vi "String Constant - Inside Nested Case Structure.vi"() -> ()   [LabVIEW 2020]
panel:
  in  "OK":bool
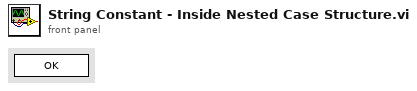
[diagram p1: front panel]
types:
  T1 = enum32{"Invalid", "Standard", "Closed", "Hidden", "Minimized", "Maximized"}
  T2 = enum32{"invalid app kind", "Development System", "Run Time System", "Student Edition", "Embedded LabVIEW", "Evaluation", "Custom"}
  T3 = cluster{"Core":cluster{"Current VI Reference":refnum<vi>, "Close Panel on Exit?":bool}, "Your Boolean data":bool}
  T4 = cluster{"Current VI Reference":refnum<vi>, "Close Panel on Exit?":bool}
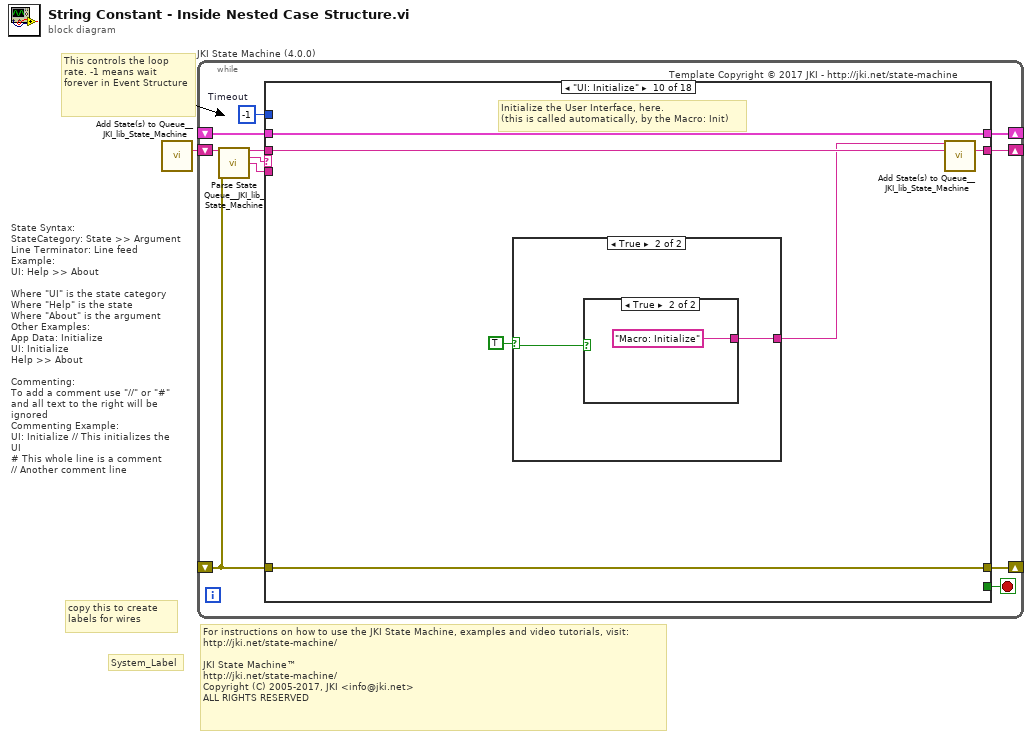
[diagram p0: block diagram]
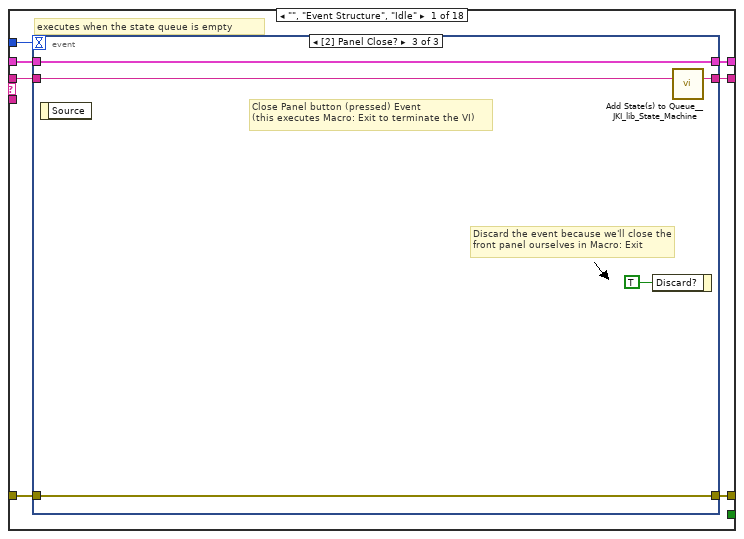
[diagram p2: hidden frame]
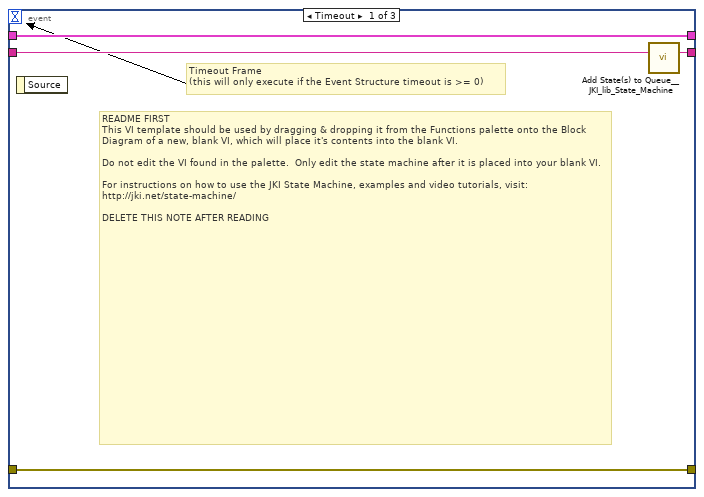
[diagram p3: hidden frame]
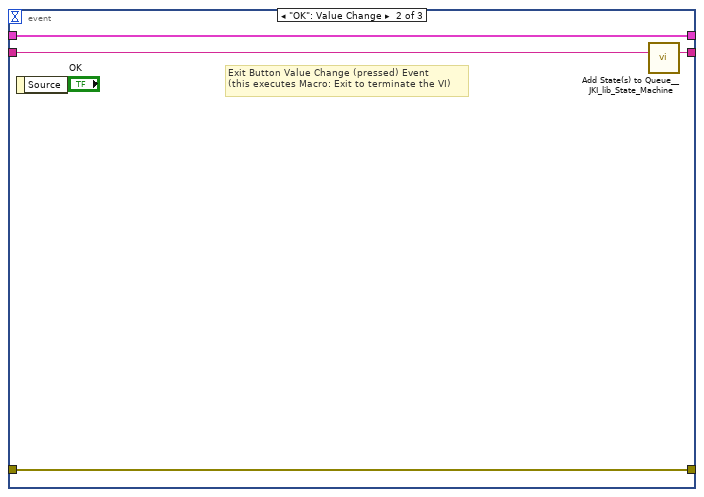
[diagram p4: hidden frame]
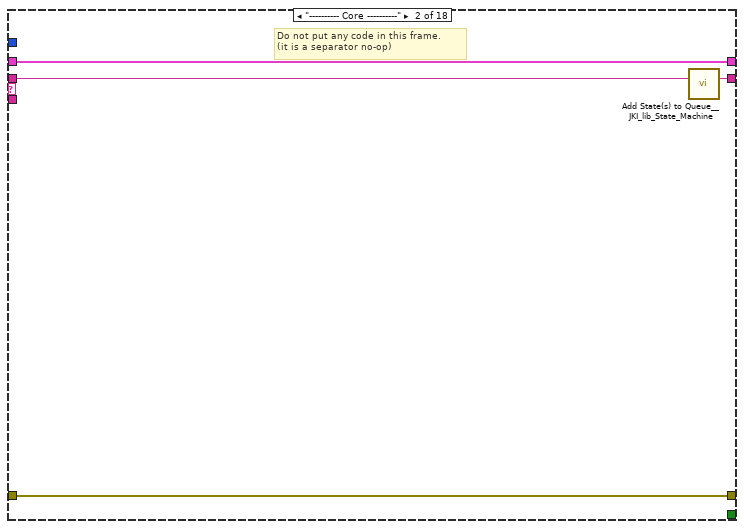
[diagram p5: hidden frame]
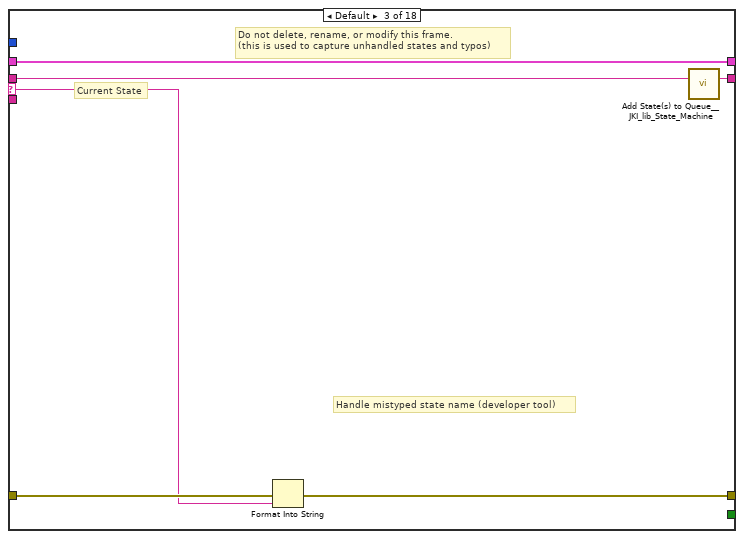
[diagram p6: hidden frame]
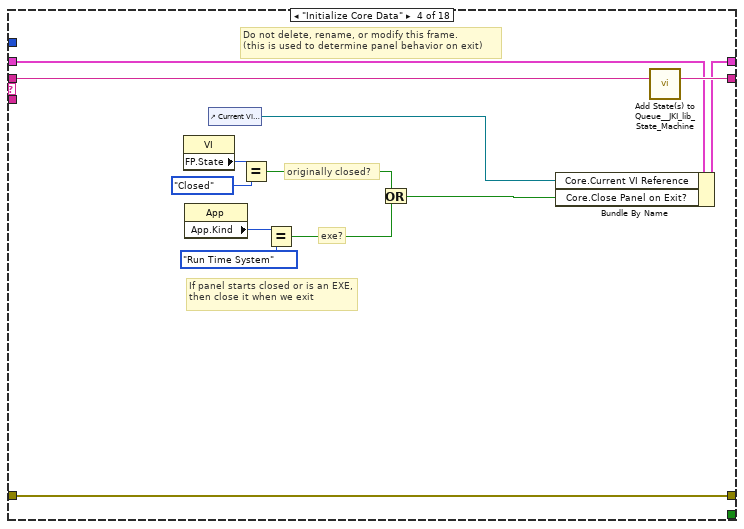
[diagram p7: hidden frame]
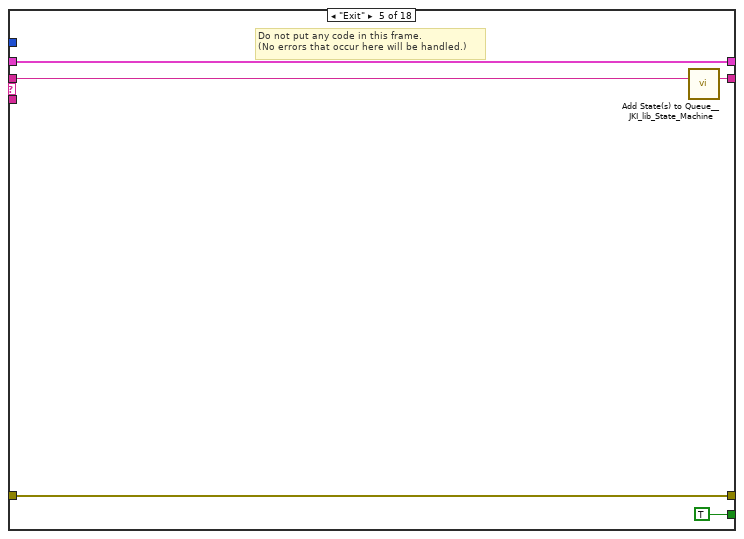
[diagram p8: hidden frame]
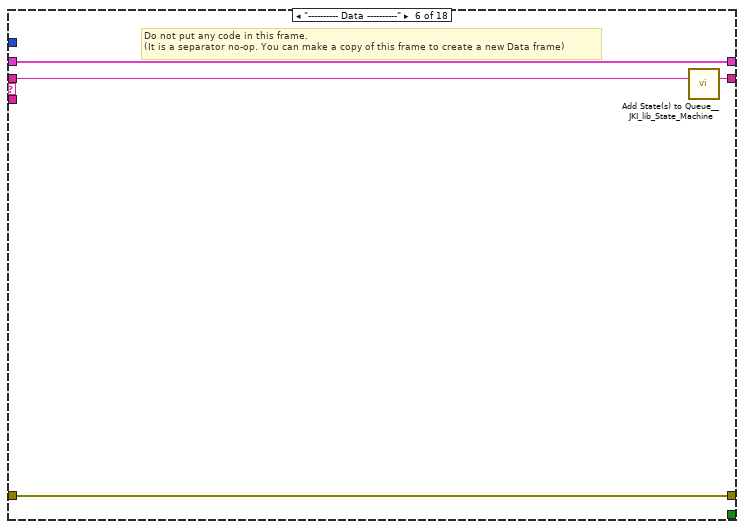
[diagram p9: hidden frame]
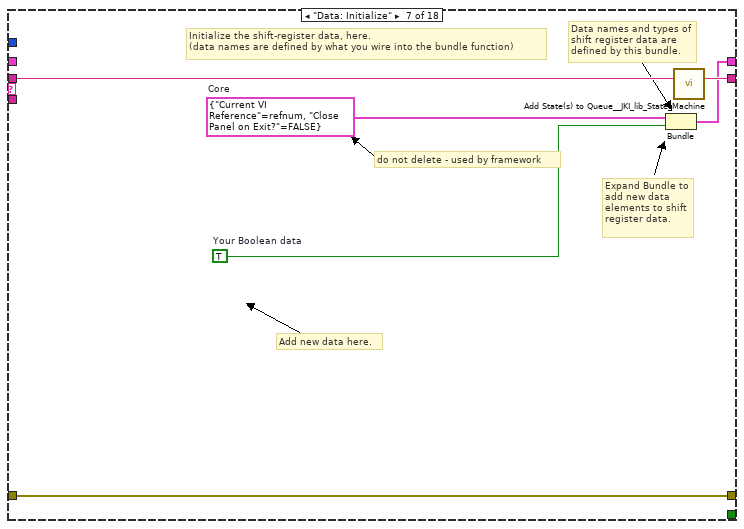
[diagram p10: hidden frame]
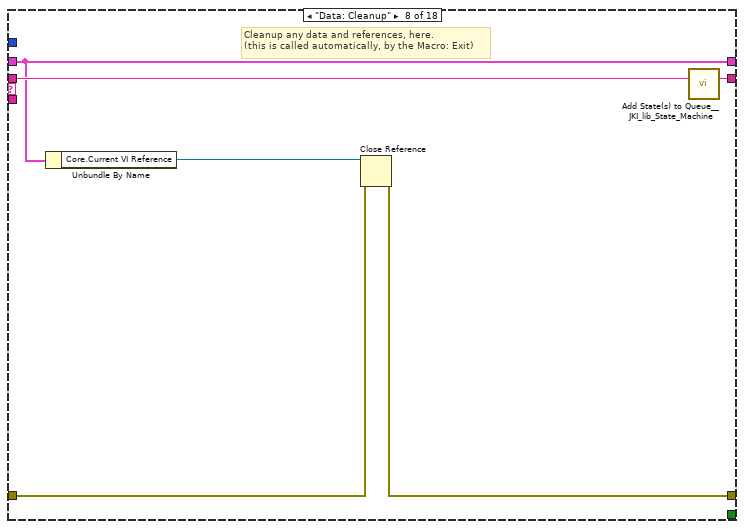
[diagram p11: hidden frame]
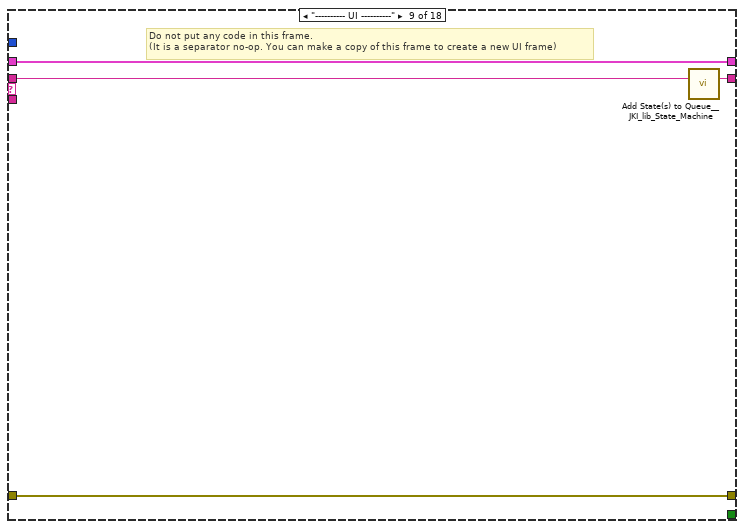
[diagram p12: hidden frame]
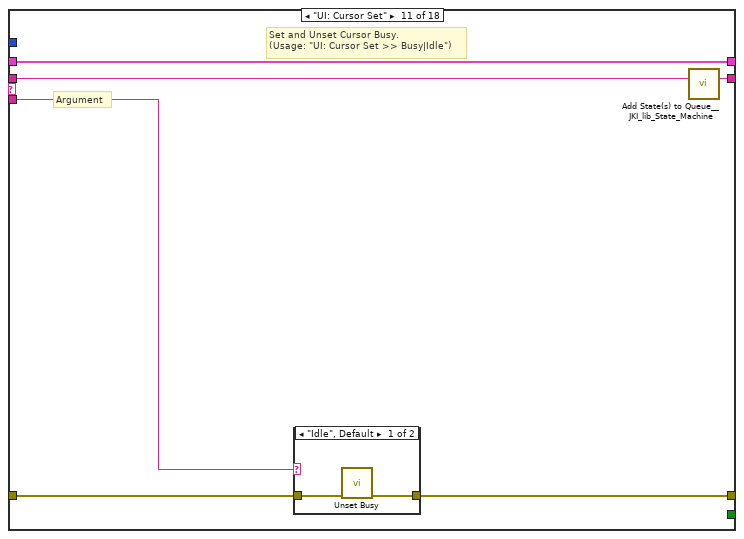
[diagram p15: hidden frame]
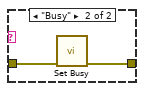
[diagram p16: hidden frame]
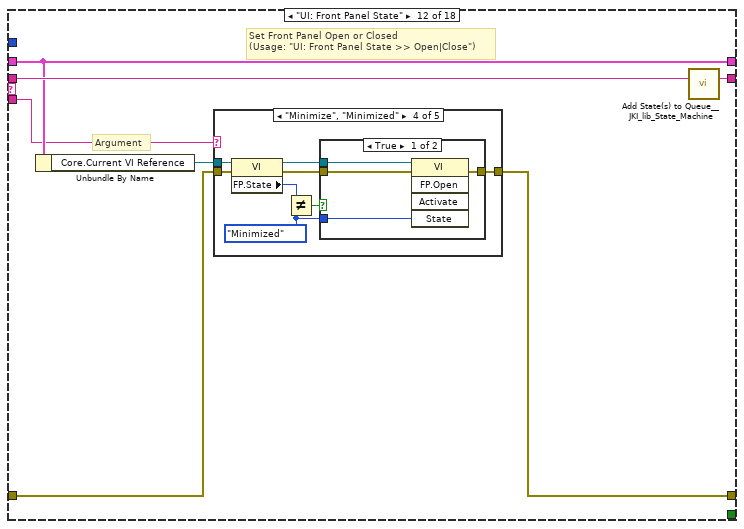
[diagram p17: hidden frame]
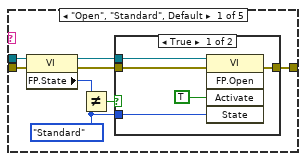
[diagram p18: hidden frame]
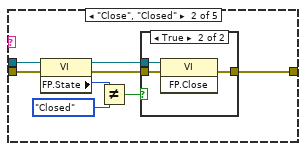
[diagram p20: hidden frame]
diagram:
  # "For instructions on how to use the JKI State Machine, examples and video tutorials, visit:\nhttp://jki.net/state-machine/\n\nJKI State Machine™\nhttp://jki.net/state-machine/\nCopyright (C) 2005-2017, JKI <info@jki.net>\nALL RIGHTS RESERVED"
  # "State Syntax:\nStateCategory: State >> Argument\nLine Terminator: Line feed\nExample:\nUI: Help >> About\n\nWhere \"UI\" is the state category\nWhere \"Help\" is the state\nWhere \"About\" is the argument\nOther Examples:\nApp Data: Initialize\nUI: Initialize\nHelp >> About\n\nCommenting:\nTo add a comment use \"//\" or \"#\" and all text to the right will be ignored\nCommenting Example:\nUI: Initialize // This initializes the UI\n# This whole line is a comment\n// Another comment line"
  # "copy this to create labels for wires"
  # "This controls the loop rate. -1 means wait forever in Event Structure"
  # "System_Label"
  n1 = call <vilib>:"Add State(s) to Queue__JKI_lib_State_Machine.vi"() -> ("States Out"=w1:string)  [unwired: 15 in]
  n2 = while "JKI State Machine (4.0.0)" {
    shift-right: [w5] -> _
    shift-left: _ -> [w4]
    shift-right: [w8] -> _
    shift-left: _ -> [w2]
    shift-right: [w7] -> _
    shift-left: w1 -> [w9]
    stop <- w6 stop-if-true
    w3 = -1  # Timeout
    # "Template Copyright © 2017 JKI - http://jki.net/state-machine"
    n3 = call <vilib>:"Parse State Queue__JKI_lib_State_Machine.vi"("State Queue"=w9, "Error In (no error)"=w2) -> ("Remaining States"=w11:string, "Current State"=w12:string, "Arguments"=w10:string)  [unwired: 11 in]
    n4 = case shown="\"UI: Initialize\"" w12 {
      selector: w12 -> [_ _ w37 _ _ _ _ _ _ _ _ _ _ _ _ _ _ _]
      tunnel: w11 -> [w19 w36 w40 w55 w60 w64 w70 w76 w80 w86 w95 w106 w175 w179 w183 w187 w191 w195]
      tunnel: w10 -> [_ _ _ _ _ _ _ _ _ _ w90 w100 _ _ _ _ _ _]
      tunnel: w4 -> [w17 w33 w38 w48 w58 w61 _ w71 w77 w84 w93 w102 w172 w176 w180 w184 w188 w192]
      tunnel: [w16 w34 w42 w52 w57 w62 w67 w72 w78 w83 w91 w103 w173 w177 w181 w185 w189 w193] -> w8
      tunnel: w2 -> [w15 w34 w41 w52 w57 w62 w67 w73 w78 w83 w92 w104 w173 w177 w181 w185 w189 w193]
      tunnel: [w18 w35 w39 w54 w59 w63 w69 w75 w79 w85 w94 w105 w174 w178 w182 w186 w190 w194] -> w7
      tunnel: [_ _ _ _ TRUE _ _ _ _ _ _ _ _ _ _ _ _ _] -> w6
      tunnel: [w14 w33 w38 w53 w58 w61 w68 w71 w77 w84 w93 w102 w172 w176 w180 w184 w188 w192] -> w5
      tunnel: w3 -> [w13 _ _ _ _ _ _ _ _ _ _ _ _ _ _ _ _ _]
      frame "", "Event Structure", "Idle" {
        # "executes when the state queue is empty"
        n5 = event shown="[2] Panel Close?" {
          selector: _ -> [_ _ _]
          dyn-events: _ -> [_ _ _]
          timeout: w13 -> [_ _ _]
          tunnel: w19 -> [w23 w27 w32]
          tunnel: [w22 w26 w31] -> w18
          tunnel: w17 -> [w20 w24 w29]
          tunnel: [w21 w25 w30] -> w16
          tunnel: w15 -> [w21 w25 w30]
          tunnel: [w20 w24 w29] -> w14
          event Timeout {
            # "README FIRST\nThis VI template should be used by dragging & dropping it from the Functions palette onto the Block Diagram of a new, blank VI, which will place it's contents into the blank VI.\n\nDo not edit the VI found in the palette.  Only edit the state machine after it is placed into your blank VI.\n\nFor instructions on how to use the JKI State Machine, examples and video tutorials, visit:\nhttp://jki.net/state-machine/\n\nDELETE THIS NOTE AFTER READING"
            # "Timeout Frame\n(this will only execute if the Event Structure timeout is >= 0)"
            n6 = event-data() -> ()  [unwired: 1 in, 1 out]
            n7 = call <vilib>:"Add State(s) to Queue__JKI_lib_State_Machine.vi"("State(s) in (\"\")"=w23) -> ("States Out"=w22:string)  [unwired: 14 in]
          }
          event "OK": Value Change {
            # "Exit Button Value Change (pressed) Event\n(this executes Macro: Exit to terminate the VI)"
            n8 = event-data() -> ()  [unwired: 1 in, 1 out]
            n9 = call <vilib>:"Add State(s) to Queue__JKI_lib_State_Machine.vi"("State(s) in (\"\")"=w27) -> ("States Out"=w26:string)  [unwired: 14 in]
          }
          event Panel Close? {
            # "Discard the event because we'll close the front panel ourselves in Macro: Exit"
            # "Close Panel button (pressed) Event\n(this executes Macro: Exit to terminate the VI)"
            n10 = event-data() -> ()  [unwired: 1 in, 1 out]
            n11 = event-data("Discard?"=TRUE) -> ()  [unwired: 1 in, 1 out]
            n12 = call <vilib>:"Add State(s) to Queue__JKI_lib_State_Machine.vi"("State(s) in (\"\")"=w32) -> ("States Out"=w31:string)  [unwired: 14 in]
          }
        }
      }
      frame "---------- Core ----------" {
        # "Do not put any code in this frame.\n(it is a separator no-op)"
        n13 = call <vilib>:"Add State(s) to Queue__JKI_lib_State_Machine.vi"("State(s) in (\"\")"=w36) -> ("States Out"=w35:string)  [unwired: 14 in]
      }
      frame Default {
        # "Current State"
        # "Do not delete, rename, or modify this frame.\n(this is used to capture unhandled states and typos)"
        # "Handle mistyped state name (developer tool)"
        n14 = Format Into String(error in=w41, w37) -> (error out=w42:errorcluster)  [unwired: 2 in, 1 out]
        n15 = call <vilib>:"Add State(s) to Queue__JKI_lib_State_Machine.vi"("State(s) in (\"\")"=w40) -> ("States Out"=w39:string)  [unwired: 14 in]
      }
      frame "Initialize Core Data" {
        # "Do not delete, rename, or modify this frame.\n(this is used to determine panel behavior on exit)"
        # "originally closed?"
        # "exe?"
        # "If panel starts closed or is an EXE, then close it when we exit"
        n16 = property class="VI"() -> ("FP.State"=w45:T1)  [unwired: 2 in, 2 out]
        n17 = property class="App"() -> ("App.Kind"=w51:T2)  [unwired: 2 in, 2 out]
        n18 = control-ref of="Current VI Reference"() -> (w46:refnum<vi>)
        n19 = Equal?(x=w45, y=T1."Closed" ("Front Panel Window:State")) -> (x = y?=w43:bool)
        n20 = Equal?(x=w51, y=T2."Run Time System" ("Application:Kind")) -> (x = y?=w49:bool)
        n21 = Or(x=w43, y=w49) -> (x .or. y?=w47:bool)
        n22 = Bundle By Name(cluster=w48, "Core.Current VI Reference"=w46, "Core.Close Panel on Exit?"=w47) -> (w53:T3)
        n23 = call <vilib>:"Add State(s) to Queue__JKI_lib_State_Machine.vi"("State(s) in (\"\")"=w55) -> ("States Out"=w54:string)  [unwired: 14 in]
      }
      frame "Exit" {
        # "Do not put any code in this frame.\n(No errors that occur here will be handled.)"
        n24 = call <vilib>:"Add State(s) to Queue__JKI_lib_State_Machine.vi"("State(s) in (\"\")"=w60) -> ("States Out"=w59:string)  [unwired: 14 in]
      }
      frame "---------- Data ----------" {
        # "Do not put any code in this frame.\n(It is a separator no-op. You can make a copy of this frame to create a new Data frame)"
        n25 = call <vilib>:"Add State(s) to Queue__JKI_lib_State_Machine.vi"("State(s) in (\"\")"=w64) -> ("States Out"=w63:string)  [unwired: 14 in]
      }
      frame "Data: Initialize" {
        w65 = T4 {"Current VI Reference"=refnum, "Close Panel on Exit?"=FALSE}  # Core
        w66 = TRUE  # Your Boolean data
        # "do not delete - used by framework"
        # "Expand Bundle to add new data elements to shift register data."
        # "Add new data here."
        # "Data names and types of shift register data are defined by this bundle."
        # "Initialize the shift-register data, here.\n(data names are defined by what you wire into the bundle function)"
        n26 = Bundle("Core"=w65, "Your Boolean data"=w66) -> (w68:T3)  [unwired: 1 in]
        n27 = call <vilib>:"Add State(s) to Queue__JKI_lib_State_Machine.vi"("State(s) in (\"\")"=w70) -> ("States Out"=w69:string)  [unwired: 14 in]
      }
      frame "Data: Cleanup" {
        # "Cleanup any data and references, here.\n(this is called automatically, by the Macro: Exit)"
        n28 = Unbundle By Name(w71) -> ("Core.Current VI Reference"=w74:refnum<vi>)
        n29 = Close Reference(reference=w74, error in (no error)=w73) -> (error out=w72:errorcluster)
        n30 = call <vilib>:"Add State(s) to Queue__JKI_lib_State_Machine.vi"("State(s) in (\"\")"=w76) -> ("States Out"=w75:string)  [unwired: 14 in]
      }
      frame "---------- UI ----------" {
        # "Do not put any code in this frame.\n(It is a separator no-op. You can make a copy of this frame to create a new UI frame)"
        n31 = call <vilib>:"Add State(s) to Queue__JKI_lib_State_Machine.vi"("State(s) in (\"\")"=w80) -> ("States Out"=w79:string)  [unwired: 14 in]
      }
      frame "UI: Initialize" {
        # "Initialize the User Interface, here.\n(this is called automatically, by the Macro: Init)"
        n32 = case shown="True" TRUE {
          selector: TRUE -> [_ w87]
          tunnel: [_ w88] -> w82
          frame False {
          }
          frame True {
            n33 = case shown="True" w87 {
              tunnel: [_ "Macro: Initialize"] -> w88
              frame False {
              }
              frame True {
              }
            }
          }
        }
        n34 = call <vilib>:"Add State(s) to Queue__JKI_lib_State_Machine.vi"("State(s) in Front (\"\")"=w82, "State(s) in (\"\")"=w86) -> ("States Out"=w85:string)  [unwired: 13 in]
      }
      frame "UI: Cursor Set" {
        # "Argument"
        # "Set and Unset Cursor Busy.\n(Usage: \"UI: Cursor Set >> Busy|Idle\")"
        n35 = case shown="\"Idle\", Default" w90 {
          tunnel: w92 -> [w97 w99]
          tunnel: [w96 w98] -> w91
          frame "Idle", Default {
            n36 = call <vilib>:"Unset Busy.vi"("error in (no error)"=w97) -> ("error out"=w96:errorcluster)  [unwired: 10 in]
          }
          frame "Busy" {
            n37 = call <vilib>:"Set Busy.vi"("error in (no error)"=w99) -> ("error out"=w98:errorcluster)  [unwired: 9 in, 1 out]
          }
        }
        n38 = call <vilib>:"Add State(s) to Queue__JKI_lib_State_Machine.vi"("State(s) in (\"\")"=w95) -> ("States Out"=w94:string)  [unwired: 14 in]
      }
      frame "UI: Front Panel State" {
        # "Argument"
        # "Set Front Panel Open or Closed\n(Usage: \"UI: Front Panel State >> Open|Close\")"
        n39 = Unbundle By Name(w102) -> ("Core.Current VI Reference"=w101:refnum<vi>)
        n40 = case shown="\"Minimize\", \"Minimized\"" w100 {
          tunnel: w104 -> [w112 w127 w138 w151 w164]
          tunnel: [w114 w128 w140 w153 w166] -> w103
          tunnel: w101 -> [w113 w125 w139 w152 w165]
          frame "Open", "Standard", Default {
            w107 = T1."Standard" ("State")
            n41 = property class="VI"(reference=w113, error in=w112) -> (reference out=w110:refnum<vi>, error out=w111:errorcluster, "FP.State"=w109:T1)
            n42 = Not Equal?(x=w109, y=w107) -> (x != y?=w108:bool)
            n43 = case shown="True" w108 {
              tunnel: [w118 w120] -> w114
              tunnel: w111 -> [w117 w120]
              tunnel: w110 -> [w116 _]
              tunnel: w107 -> [w115 _]
              frame True {
                n44 = invoke class="VI" method="FP.Open"(reference=w116, error in=w117, "Activate"=TRUE, "State"=w115) -> (error out=w118:errorcluster)  [unwired: 1 in, 4 out]
              }
              frame False {
              }
            }
          }
          frame "Close", "Closed" {
            n45 = property class="VI"(reference=w125, error in=w127) -> (reference out=w124:refnum<vi>, error out=w126:errorcluster, "FP.State"=w122:T1)
            n46 = Not Equal?(x=w122, y=T1."Closed" ("Front Panel Window:State")) -> (x != y?=w121:bool)
            n47 = case shown="True" w121 {
              tunnel: [w129 w132] -> w128
              tunnel: w126 -> [w129 w131]
              tunnel: w124 -> [_ w130]
              frame False {
              }
              frame True {
                n48 = invoke class="VI" method="FP.Close"(reference=w130, error in=w131) -> (error out=w132:errorcluster)  [unwired: 1 in, 2 out]
              }
            }
          }
          frame "Hidden", "Hide" {
            w133 = T1."Hidden" ("State")
            n49 = property class="VI"(reference=w139, error in=w138) -> (reference out=w136:refnum<vi>, error out=w137:errorcluster, "FP.State"=w135:T1)
            n50 = Not Equal?(x=w135, y=w133) -> (x != y?=w134:bool)
            n51 = case shown="True" w134 {
              tunnel: [w144 w145] -> w140
              tunnel: w137 -> [w143 w145]
              tunnel: w136 -> [w142 _]
              tunnel: w133 -> [w141 _]
              frame True {
                n52 = invoke class="VI" method="FP.Open"(reference=w142, error in=w143, "State"=w141) -> (error out=w144:errorcluster)  [unwired: 2 in, 4 out]
              }
              frame False {
              }
            }
          }
          frame "Minimize", "Minimized" {
            w146 = T1."Minimized" ("State")
            n53 = property class="VI"(reference=w152, error in=w151) -> (reference out=w149:refnum<vi>, error out=w150:errorcluster, "FP.State"=w148:T1)
            n54 = Not Equal?(x=w148, y=w146) -> (x != y?=w147:bool)
            n55 = case shown="True" w147 {
              tunnel: [w157 w158] -> w153
              tunnel: w150 -> [w156 w158]
              tunnel: w149 -> [w155 _]
              tunnel: w146 -> [w154 _]
              frame True {
                n56 = invoke class="VI" method="FP.Open"(reference=w155, error in=w156, "State"=w154) -> (error out=w157:errorcluster)  [unwired: 2 in, 4 out]
              }
              frame False {
              }
            }
          }
          frame "Maximize", "Maximized" {
            w159 = T1."Maximized" ("State")
            n57 = property class="VI"(reference=w165, error in=w164) -> (reference out=w162:refnum<vi>, error out=w163:errorcluster, "FP.State"=w161:T1)
            n58 = Not Equal?(x=w161, y=w159) -> (x != y?=w160:bool)
            n59 = case shown="True" w160 {
              tunnel: [w170 w171] -> w166
              tunnel: w163 -> [w169 w171]
              tunnel: w162 -> [w168 _]
              tunnel: w159 -> [w167 _]
              frame True {
                n60 = invoke class="VI" method="FP.Open"(reference=w168, error in=w169, "State"=w167) -> (error out=w170:errorcluster)  [unwired: 2 in, 4 out]
              }
              frame False {
              }
            }
          }
        }
        n61 = call <vilib>:"Add State(s) to Queue__JKI_lib_State_Machine.vi"("State(s) in (\"\")"=w106) -> ("States Out"=w105:string)  [unwired: 14 in]
      }
      frame "---------- Macro ----------" {
        # "Do not put any code in this frame.\n(It is a separator no-op. You can make a copy of this frame to create a new Macro frame)"
        n62 = call <vilib>:"Add State(s) to Queue__JKI_lib_State_Machine.vi"("State(s) in (\"\")"=w175) -> ("States Out"=w174:string)  [unwired: 14 in]
      }
      frame "Macro: Initialize" {
        # "Initialization Macro\n(This is called once, when the VI starts)"
        n63 = call <vilib>:"Add State(s) to Queue__JKI_lib_State_Machine.vi"("State(s) in (\"\")"=w179) -> ("States Out"=w178:string)  [unwired: 14 in]
      }
      frame "Macro: Exit" {
        # "Exit Macro\n(This is called once, when the VI exits)"
        n64 = call <vilib>:"Add State(s) to Queue__JKI_lib_State_Machine.vi"("State(s) in (\"\")"=w183) -> ("States Out"=w182:string)  [unwired: 14 in]
      }
      frame "---------- New Category ----------" {
        # "Template Separator\n(You can make a copy of, or modify, this frame)"
        n65 = call <vilib>:"Add State(s) to Queue__JKI_lib_State_Machine.vi"("State(s) in (\"\")"=w187) -> ("States Out"=w186:string)  [unwired: 14 in]
      }
      frame "New Category: 1" {
        # "Your code here.\n(You can make a copy of, or modify, this frame)"
        n66 = call <vilib>:"Add State(s) to Queue__JKI_lib_State_Machine.vi"("State(s) in (\"\")"=w191) -> ("States Out"=w190:string)  [unwired: 14 in]
      }
      frame "New Category: 2" {
        # "Your code here.\n(You can make a copy of, or modify, this frame)"
        n67 = call <vilib>:"Add State(s) to Queue__JKI_lib_State_Machine.vi"("State(s) in (\"\")"=w195) -> ("States Out"=w194:string)  [unwired: 14 in]
      }
    }
  }
